vi "GetConfigurationBasePath.vi"(8 "ErrorIn":errorcluster, 11 "ReferenceIn":refnum<class "AppConfigJSON.lvclass">) -> (0 "ErrorOut":errorcluster, 1 "ApplicationBasePath":path, 3 "ReferenceOut":refnum<class "AppConfigJSON.lvclass">)   [LabVIEW 2021, in "AppConfigJSON.lvclass"]
uses:
  AppConfigJSON.lvclass
  AppConfigJSON.lvclass/AppConfigJSON.ctl
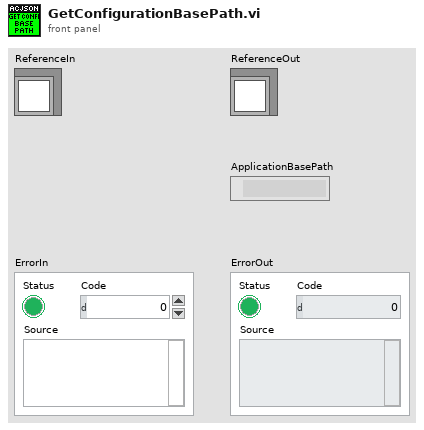
[diagram p1: front panel]
types:
  T1 = typedef "AppConfigJSON.lvclass/ObjectAttributes.ctl" = cluster{"Name":string, "ConfigFilePath":path, "Objects":T2[], "ApplicationBasePath":path, "ObjectName":string}
  T2 = typedef "IApplicationConfiguration.lvclass/ObjectDataDetails.ctl" = cluster{"ObjectName":string, "ObjectType":string, "Interfaces":T3[]}
  T3 = typedef "IApplicationConfiguration.lvclass/ObjectData.ctl" = cluster{"Label":string, "ObjectName":string, "Type":string}
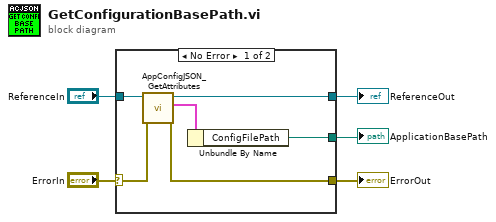
[diagram p0: block diagram]
diagram:
  n1 = case shown="No Error" "ErrorIn" {
    selector: "ErrorIn" -> [w11 w13]
    tunnel: [w10 w13] -> w4
    tunnel: [w7 w12] -> w2
    tunnel: "ReferenceIn" -> [w8 w12]
    tunnel: [w6 _] -> w1
    frame No Error {
      n2 = call "AppConfigJSON_GetAttributes.vi"("ErrorIn"=w11, "ReferenceIn"=w8) -> ("ErrorOut"=w10:errorcluster, "Data"=w9:T1, "ReferenceOut"=w7:refnum<class "AppConfigJSON.lvclass">)  [unwired: 6 in, 1 out]
      n3 = Unbundle By Name(w9) -> ("ConfigFilePath"=w6:path)
    }
    frame Error {
    }
  }
  "ErrorOut" <- w4
  "ReferenceOut" <- w2
  "ApplicationBasePath" <- w1
